vi "Robot Global Data.vi"() -> ()   [LabVIEW 2015]
doc: "This global VI can contain as many global variables as you need. Place a control on the panel, give it a good name. To read or write to it from a VI, drag the icon to the diagram of that VI. You can also drag from the project. Click on the node to change which global you access. You shouldn't have multiple locations writing to a global or it will cause a race-condition."
uses:
  <vilib>/Rock Robotics/WPI/Camera/WPI_CameraImageSize.ctl
  <vilib>/Rock Robotics/WPI/DriverStation/WPI_DriverStationRobotMode2.ctl
  shooter/shooter.lvclass
  drive/drive.lvclass
  intake/intake.lvclass
  arm/arm.lvclass
panel:
  in  "arm":refnum<class "arm.lvclass">
  in  "intake":refnum<class "intake.lvclass">
  in  "drive":refnum<class "drive.lvclass">
  in  "shooter":refnum<class "shooter.lvclass">
  out "Shooter Disable":bool
  in  "poses 2":cluster{"theta":dbl, "x":dbl, "y":dbl}[](array[cluster])
  in  "Arm Angle":dbl
  out "Intake Disable":bool
  out "Shoot tele":bool
  in  "Target Heading":dbl
  in  "poses":cluster{"theta":dbl}[](array[cluster])
  out "Pot Value Right":dbl
  out "Pot Value":dbl
  out "Automated Aim":bool
  out "Doing auto in tele":bool
  out "Arm Disable":bool
  out "Drive Disable":bool
  out "CDF Tele":bool
  out "Porticullis Tele":bool
  out "mechanismEncoder":dbl
  out "Collapse Arm Button":bool
  out "Extend Arm Button":bool
  in  "Robot Mode":T1
  in  "image size":T2=enum."320x240"
  in  "Enable Vision":bool
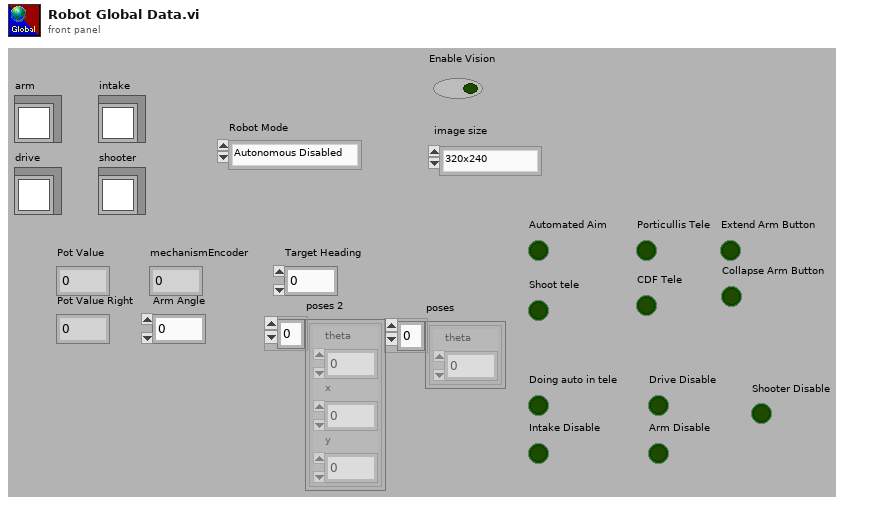
[diagram p1: front panel]
types:
  T1 = typedef "WPI_DriverStationRobotMode2.ctl" = enum16{"Autonomous Disabled", "Autonomous Enabled", "Teleop Disabled", "Teleop Enabled", "Disconnected", "Finish", "Test Disabled", "Test Enabled", "Emergency Stopped"}
  T2 = typedef "WPI_CameraImageSize.ctl" = enum16{"640x480", "320x240", "160x120", "Custom"}
diagram:
